vi "ex14-11.vi"() -> ()   [LabVIEW 2014]
panel:
  out "X AND Y":dbl
  in  "Y":dbl
  in  "X":dbl
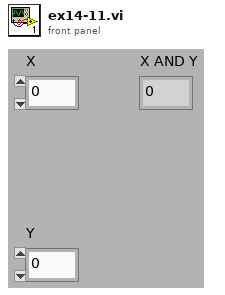
[diagram p1: front panel]
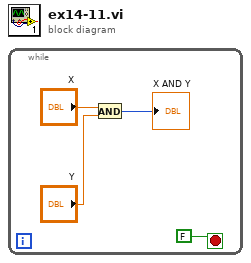
[diagram p0: block diagram]
diagram:
  n1 = while {
    stop <- FALSE stop-if-true
    n2 = And(x="X", y="Y") -> (x .and. y?=→"X AND Y":i32)
  }
